vi "Modbus Main Page.vi"(8 "error in (no error)":errorcluster, 11 "Node Ptr":T1 format="%.0x") -> (0 "error out":errorcluster)   [LabVIEW 2014, in "Modbus System Explorer.lvlib"]
uses:
  Modbus System Explorer.lvlib
  <vilib>/NI Veristand/Custom Device API/Custom Device Item Ref.ctl
  Glyphs/Modbus Property Names.vi
  <vilib>/NI Veristand/Custom Device API/Get Item Property (String).vi
  <vilib>/NI Veristand/Custom Device API/Get Item Property (Path).vi
  <vilib>/NI Veristand/Custom Device API/Custom Device API.lvlib
  Shared/Modbus Shared.lvlib
panel:
  out "Version":string
  out "Last File content":string
  out "MD5 Hash":string
  in  "File Path":path
  in  "Load_Reload File":bool
  in  "Header":cluster{"Section Name":string}={"Section Name"="Modbus Custom Device Item Settings"}
  in  "Description":string
  in  "Name":string
  # "Modbus Configuration"
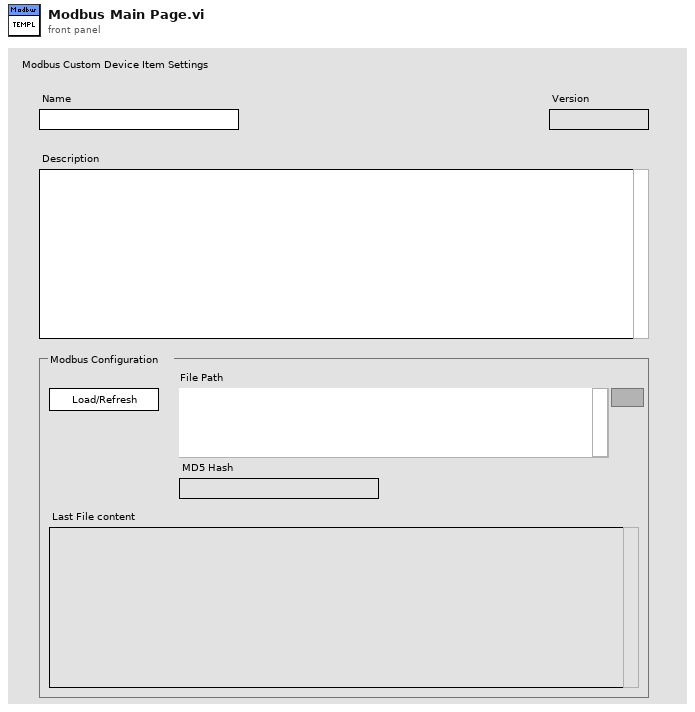
[diagram p1: front panel]
types:
  T1 = typedef "Custom Device API.lvlib/Custom Device Item Ref.ctl" = u64
  T2 = typedef "Custom Device API.lvlib/Custom Device Item Info.ctl" = cluster{"Name":string, "Is Channel":bool, "GUID":string, "Is Waveform":bool}
  T3 = typedef "Custom Device API.lvlib/Custom Device Commands.ctl" = enum16{"Default", "Item renamed", "Shutdown", "Dynamic button pressed"}
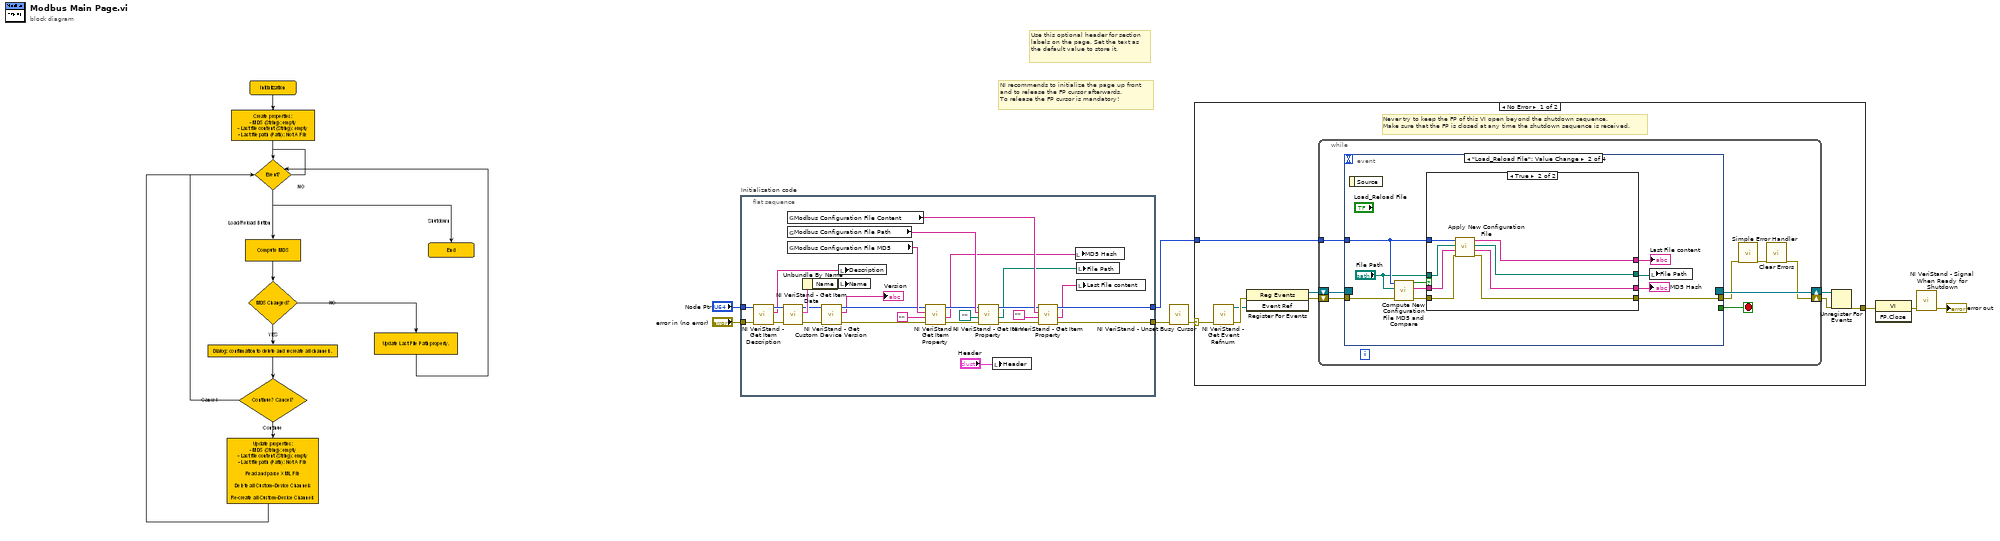
[diagram p0: block diagram]
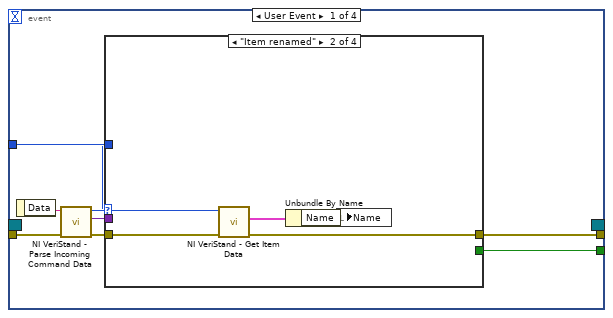
[diagram p2: hidden frame]
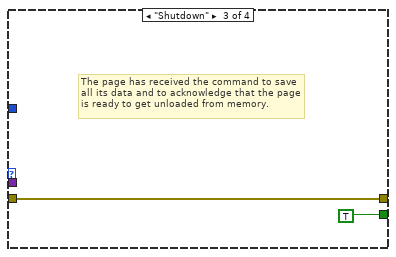
[diagram p4: hidden frame]
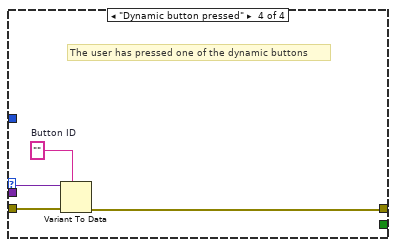
[diagram p5: hidden frame]
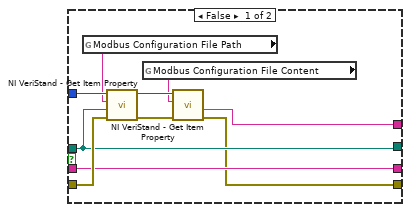
[diagram p6: hidden frame]
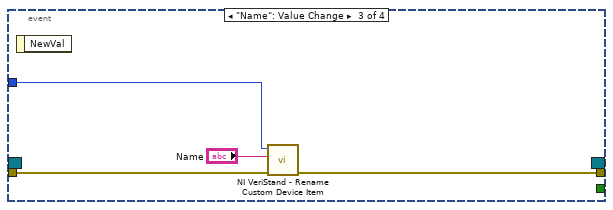
[diagram p7: hidden frame]
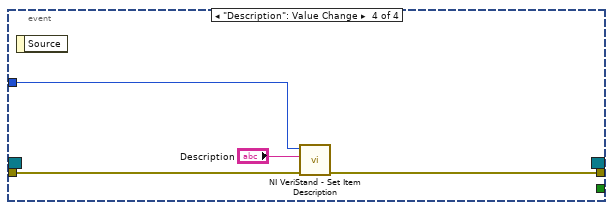
[diagram p8: hidden frame]
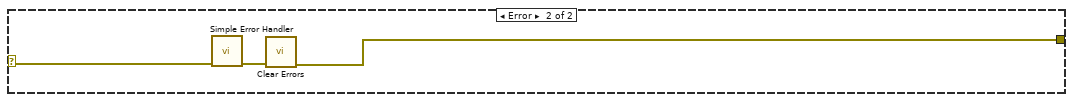
[diagram p9: hidden frame]
diagram:
  # "Use this optional header for section labels on the page. Set the text as the default value to store it."
  # "NI recommends to initialize the page up front\nand to release the FP cursor afterwards.\nTo release the FP cursor is mandatory!"
  n1 = flat-sequence "Initialization code" {
    tunnel: "error in (no error)" -> [w35]
    tunnel: "Node Ptr" -> [w34]
    tunnel: [w21] -> w4
    tunnel: [w22] -> w1
    frame #0 {
      n2 = call <vilib>:"NI VeriStand - Get Item Description.vi"("error in (no error)"=w35, "Item Ref in"=w34) -> ("error out"=w32:errorcluster, "Description"=w33:string, "Item Ref out"=w36:T1)  [unwired: 7 out]
      n3 = call <vilib>:"NI VeriStand - Get Item Data.vi"("error in (no error)"=w32, "Item Ref in"=w36) -> ("error out"=w13:errorcluster, "Item Info"=w31:T2, "Item Ref out"=w14:T1)  [unwired: 7 out]
      n4 = global read "Modbus Property Names.vi" "Modbus Configuration File Content"() -> (w29:string)
      n5 = global read "Modbus Property Names.vi" "Modbus Configuration File Path"() -> (w26:string)
      n6 = global read "Modbus Property Names.vi" "Modbus Configuration File MD5"() -> (w23:string)
      n7 = Unbundle By Name(w31) -> ("Name"=w30:string)
      n8 = call <vilib>:"NI VeriStand - Get Custom Device Version.vi"("error in (no error)"=w13, "Device Ref in"=w14) -> ("error out"=w11:errorcluster, "Value"=→"Version":string, "Device Ref out"=w12:T1)  [unwired: 7 in]
      n9 = local write "Description"(w33) -> ()
      n10 = local write "Name"(w30) -> ()
      n11 = call-poly <vilib>:"NI VeriStand - Get Item Property.vi"("error in (no error)"=w11, "Default Value"="", "Property Name"=w23, "Item Ref in"=w12) -> ("error out"=w24:errorcluster, "Value"=w17:string, "Item Ref out"=w25:T1)  [unwired: 4 in, 1 out]
      n12 = call-poly <vilib>:"NI VeriStand - Get Item Property.vi"("error in (no error)"=w24, "Default Value"=path "", "Property Name"=w26, "Item Ref in"=w25) -> ("error out"=w28:errorcluster, "Value"=w16:path, "Item Ref out"=w27:T1)  [unwired: 4 in, 1 out]
      n13 = local write "Header"("Header") -> ()
      n14 = call-poly <vilib>:"NI VeriStand - Get Item Property.vi"("error in (no error)"=w28, "Default Value"="", "Property Name"=w29, "Item Ref in"=w27) -> ("error out"=w21:errorcluster, "Value"=w15:string, "Item Ref out"=w22:T1)  [unwired: 4 in, 1 out]
      n15 = local write "MD5 Hash"(w17) -> ()
      n16 = local write "File Path"(w16) -> ()
      n17 = local write "Last File content"(w15) -> ()
    }
  }
  n18 = call <vilib>:"NI VeriStand - Unset Busy Cursor.vi"("error in (no error)"=w4) -> ("error out"=w3:errorcluster)  [unwired: 10 out]
  n19 = case shown="No Error" w3 {
    selector: w3 -> [w37 w112]
    tunnel: [w42 w110] -> w8
    tunnel: w1 -> [w38 _]
    frame No Error {
      # "Never try to keep the FP of this VI open beyond the shutdown sequence.\nMake sure that the FP is closed at any time the shutdown sequence is received."
      n20 = call <vilib>:"NI VeriStand - Get Event Refnum.vi"("error in (no error)"=w37) -> ("error out"=w45:errorcluster, "Event Ref"=w41:refnum<user-event>)  [unwired: 9 out]
      n21 = register-events(error in=w45, w41) -> (reference out=w39:refnum<event-registration>, error out=w40:errorcluster)  [unwired: 1 in]
      n22 = while {
        tunnel: w38 -> [w49]
        shift-right: [w46] -> w43
        shift-left: w40 -> [w52]
        shift-right: [w53] -> w44
        shift-left: w39 -> [w51]
        stop <- w50 stop-if-true
        n23 = event shown="[1] \"Load_Reload File\": Value Change" {
          selector: w51 -> [_ _ _ _]
          dyn-events: [_ _ _ _] -> w53
          timeout: _ -> [_ _ _ _]
          tunnel: w52 -> [w61 w83 w105 w108]
          tunnel: [w57 _ _ _] -> w50
          tunnel: [w56 w75 w104 w107] -> w48
          tunnel: w49 -> [w55 w80 w103 w109]
          event User Event {
            n24 = event-data() -> ("Data"=w60:string)  [unwired: 1 out]
            n25 = call <vilib>:"NI VeriStand - Parse Incoming Command Data.vi"("error in (no error)"=w61, "Incoming data"=w60) -> ("error out"=w59:errorcluster, "Outgoing data"=w54:variant, "Action"=w58:T3)  [unwired: 7 out]
            n26 = case shown="\"Item renamed\"" w58 {
              tunnel: w59 -> [w62 w67 w68 w73]
              tunnel: [_ _ TRUE _] -> w57
              tunnel: [w62 w64 w68 w70] -> w56
              tunnel: w55 -> [_ w66 _ _]
              tunnel: w54 -> [_ _ _ w72]
              frame "Default", Default {
              }
              frame "Item renamed" {
                n27 = call <vilib>:"NI VeriStand - Get Item Data.vi"("error in (no error)"=w67, "Item Ref in"=w66) -> ("error out"=w64:errorcluster, "Item Info"=w65:T2)  [unwired: 8 out]
                n28 = Unbundle By Name(w65) -> ("Name"=w63:string)
                n29 = local write "Name"(w63) -> ()
              }
              frame "Shutdown" {
                # "The page has received the command to save all its data and to acknowledge that the page is ready to get unloaded from memory."
              }
              frame "Dynamic button pressed" {
                w71 = ""  # Button ID
                # "The user has pressed one of the dynamic buttons"
                n30 = Variant To Data(error in=w73, type=w71, Variant=w72) -> (error out=w70:errorcluster)  [unwired: 1 out]
              }
            }
          }
          event "Load_Reload File": Value Change {
            n31 = event-data() -> ()  [unwired: 2 out]
            n32 = call "Compute New Configuration File MD5 and Compare.vi"("error in (no error)"=w83, "New Path File"="File Path", "CD Ref In"=w80) -> ("error out"=w81:errorcluster, "MD5 message-digest"=w78:string, "MD5 Changed?"=w82:bool)  [unwired: 6 in]
            n33 = case shown="True" w82 {
              tunnel: w81 -> [w92 w101]
              tunnel: w80 -> [w93 w100]
              tunnel: "File Path" -> [w91 w99]
              tunnel: w78 -> [w90 w94]
              tunnel: [w91 w97] -> w77
              tunnel: [w90 w98] -> w76
              tunnel: [w85 w95] -> w75
              tunnel: [w86 w96] -> w74
              frame False {
                n34 = global read "Modbus Property Names.vi" "Modbus Configuration File Path"() -> (w84:string)
                n35 = call-poly <vilib>:"NI VeriStand - Get Item Property.vi"("error in (no error)"=w92, "Default Value"=w91, "Property Name"=w84, "Item Ref in"=w93) -> ("error out"=w88:errorcluster, "Item Ref out"=w89:T1)  [unwired: 4 in, 2 out]
                n36 = global read "Modbus Property Names.vi" "Modbus Configuration File Content"() -> (w87:string)
                n37 = call-poly <vilib>:"NI VeriStand - Get Item Property.vi"("error in (no error)"=w88, "Property Name"=w87, "Item Ref in"=w89) -> ("error out"=w85:errorcluster, "Value"=w86:string)  [unwired: 5 in, 2 out]
              }
              frame True {
                n38 = call "Apply New Configuration File.vi"("error in (no error)"=w101, "MD5 Hash In"=w94, "File Path In"=w99, "CD Ref In"=w100) -> ("error out"=w95:errorcluster, "MD5 Hash Out"=w98:string, "File Path Out"=w97:path, "Last File content"=w96:string)  [unwired: 4 in]
              }
            }
            "MD5 Hash" <- w76
            "Last File content" <- w74
            n39 = local write "File Path"(w77) -> ()
          }
          event "Name": Value Change {
            n40 = event-data() -> ()  [unwired: 2 out]
            n41 = call <vilib>:"NI VeriStand - Rename Custom Device Item.vi"("error in (no error)"=w105, "New Name"="Name", "Item Ref in"=w103) -> ("error out"=w104:errorcluster)  [unwired: 1 in, 7 out]
          }
          event "Description": Value Change {
            n42 = event-data() -> ()  [unwired: 2 out]
            n43 = call <vilib>:"NI VeriStand - Set Item Description.vi"("error in (no error)"=w108, "Description"="Description", "Item Ref in"=w109) -> ("error out"=w107:errorcluster)  [unwired: 8 out]
          }
        }
        n44 = call <vilib>:"Simple Error Handler.vi"("error in (no error)"=w48) -> ("error out"=w47:errorcluster)  [unwired: 1 in, 7 out]
        n45 = call <vilib>:"Clear Errors.vi"("error in (no error)"=w47) -> ("error out"=w46:errorcluster)  [unwired: 1 in, 5 out]
      }
      n46 = Unregister For Events(event registration refnum=w44, error in=w43) -> (error out=w42:errorcluster)
    }
    frame Error {
      n47 = call <vilib>:"Simple Error Handler.vi"("error in (no error)"=w112) -> ("error out"=w111:errorcluster)  [unwired: 1 in, 7 out]
      n48 = call <vilib>:"Clear Errors.vi"("error in (no error)"=w111) -> ("error out"=w110:errorcluster)  [unwired: 1 in, 5 out]
    }
  }
  n49 = invoke class="VI" method="FP.Close"(error in=w8) -> (error out=w7:errorcluster)  [unwired: 2 in, 2 out]
  n50 = call <vilib>:"NI VeriStand - Signal When Ready for Shutdown.vi"("error in (no error)"=w7) -> ("error out"=→"error out":errorcluster)  [unwired: 10 out]
